vi "playback.vi"() -> ()   [LabVIEW 2012]
doc: "This VI will initialize the FPGA VI and read a user-defined number of samples from a DMA FIFO. When the data acquisition is complete this VI will read status information from the FPGA VI.\n\nFollow these instructions to run the VI.\n\n1. Select your RIO device from the dropdown.\n2. Set the sample period, number of samples to acquire per channel, and DMA block read size. \n\nNote: the block read size should be set to balance load on the host processor and the update rate of the user interface. A small block read size will update the user interface more often but will result in a higher load on the host processor."
uses:
  <vilib>/Analysis/3filter.llb/Butterworth Filter (DBL).vi
  <vilib>/Analysis/NI_AALBase.lvlib
  <vilib>/Analysis/NI_AALPro.lvlib
panel:
  in  "Filename":path=path "tdms"
  in  "Next Signal":bool
  in  "threshold ratio":dbl=3.0
  out "Sidemove":dbl
  out "Forward":dbl
  out "Threshold 3":dbl
  out "Threshold 2":dbl
  out "Threshold 1":dbl
  out "noise index":dbl[](array[numeric])
  out "Threshold 0":dbl
  out "Amplitude Spectrum":waveform(dbl)(graph)
  out "bad signal?":bool
  in  "Min Starting Index":i32=7000
  in  "Portion Duration":i32=1000
  out "amplitude 3":dbl
  out "amplitude 2":dbl
  out "amplitude 1":dbl
  out "amplitude 0":dbl
  in  "noise min":dbl=0.001
  out "Index 3":dbl
  out "Index 2":dbl
  out "Index 1":dbl
  out "Index 0":dbl
  in  "Send to ROS":bool
  out "ROS  Error":bool
  out "dt1":dbl
  out "dt2":dbl
  out "dt3":dbl
  out "pitch":dbl
  out "yaw":dbl
  out "z":dbl
  out "y":dbl
  out "x":dbl
  in  "Mode":T1(ring)=enum."Use Far Field"
  in  "Altitude":dbl=2.0
  in  "Display Filtered Signal":bool=TRUE
  out "Ratio at Index (%)":dbl
  out "Selected Index":i32
  in  "Threshold":dbl=0.1
  in  "low cutoff freq: fl":dbl=20000.0
  in  "high cutoff freq: fh":dbl=30000.0
  out "Yaw Chart":dbl(graph)
  out "Ch0 Signal":dbl[](graph)
  out "Extracted signal":dbl[][](graph)
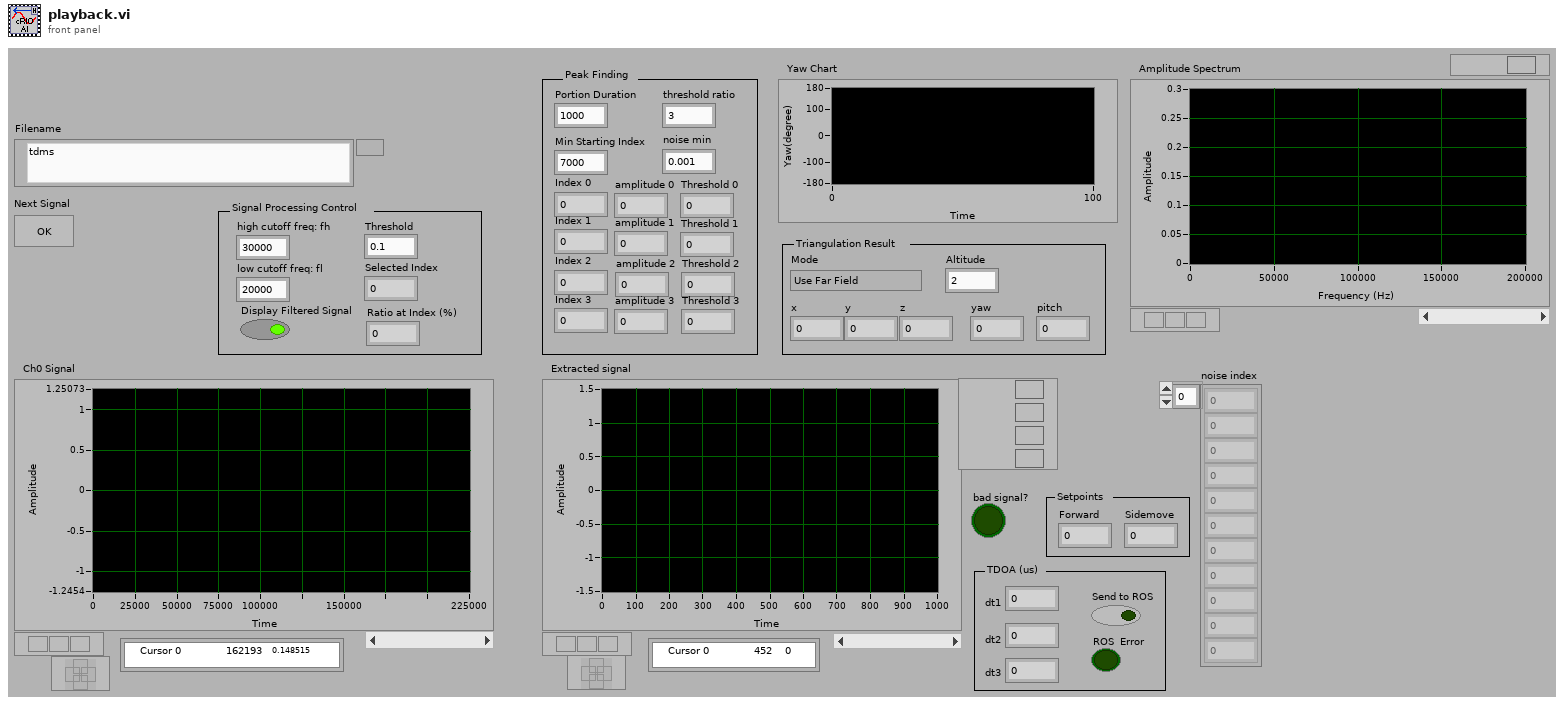
[diagram p1: front panel]
types:
  T1 = enum16{"Use Near Field", "Use Far Field", "Far Field with 3 hydrophones"}
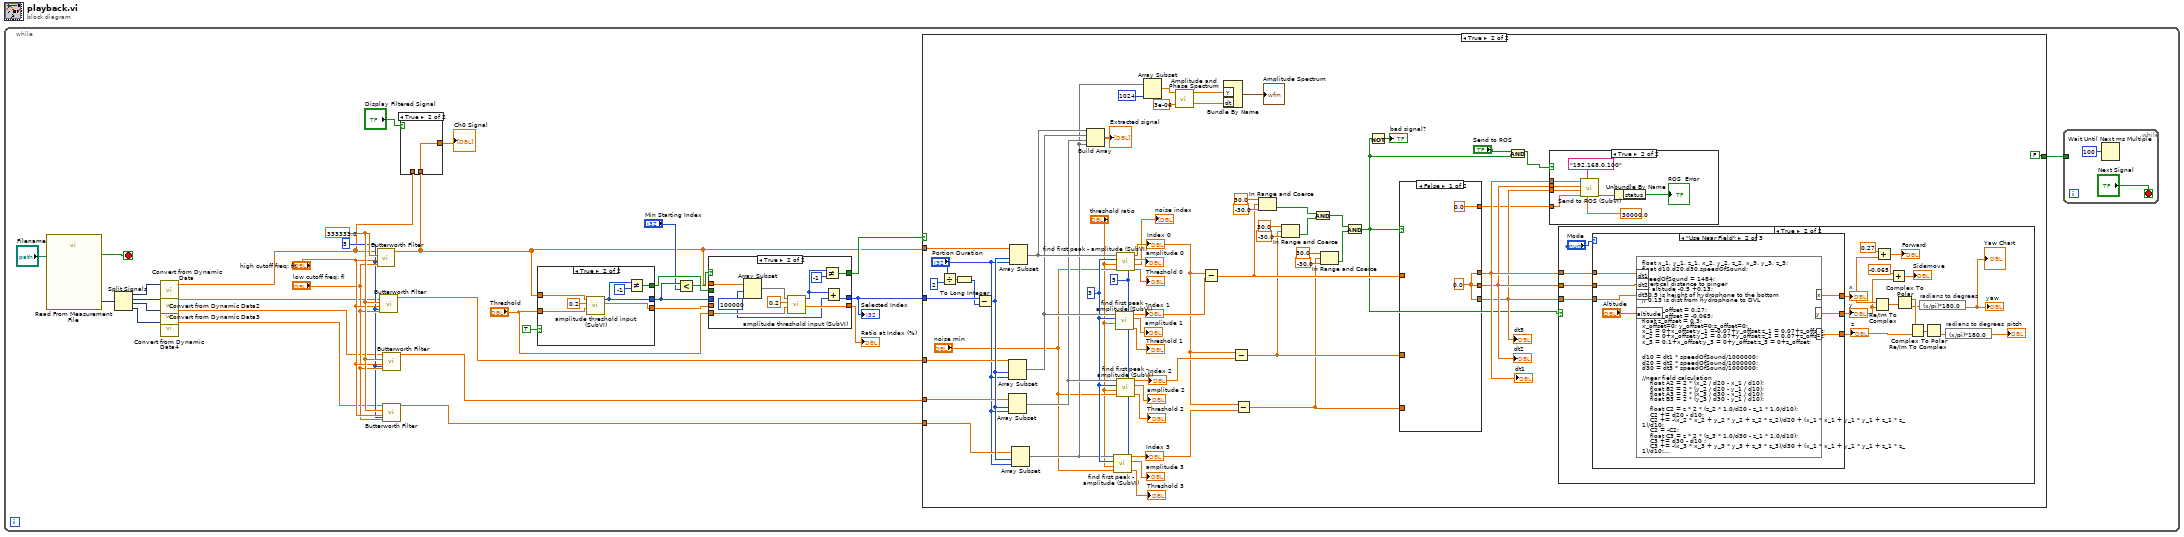
[diagram p0: block diagram]
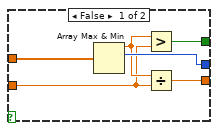
[diagram p4: hidden frame]
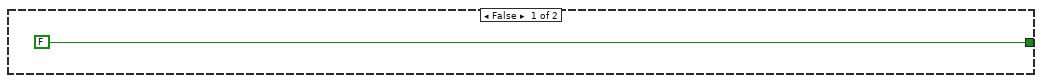
[diagram p5: hidden frame]
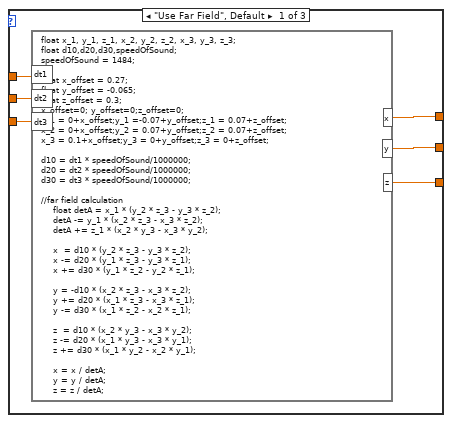
[diagram p7: hidden frame]
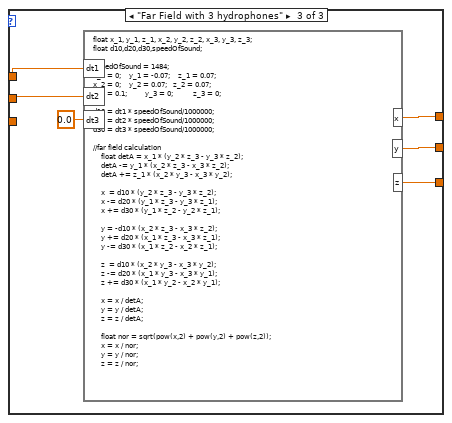
[diagram p8: hidden frame]
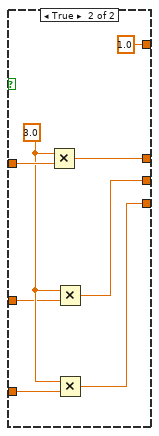
[diagram p10: hidden frame]
diagram:
  n1 = while {
    stop <- w5 stop-if-true
    w17 = 5
    w23 = 333333.0
    n2 = call "Read From Measurement File"("Filename"="Filename") -> ("Signals"=w10:dynamicdata, "EOF?"=w5:bool)  [unwired: 5 in, 4 out]
    n3 = Split Signals(w10) -> (w14:dynamicdata, w13:dynamicdata, w12:dynamicdata, w11:dynamicdata)  [unwired: 4 in]
    n4 = call "Convert from Dynamic Data"("Dynamic Data Type"=w14) -> ("Array"=w9:dbl[])  [unwired: 3 in]
    n5 = call "Convert from Dynamic Data2"("Dynamic Data Type"=w13) -> ("Array"=w8:dbl[])  [unwired: 3 in]
    n6 = call "Convert from Dynamic Data3"("Dynamic Data Type"=w12) -> ("Array"=w6:dbl[])  [unwired: 3 in]
    n7 = call "Convert from Dynamic Data4"("Dynamic Data Type"=w11) -> ("Array"=w7:dbl[])  [unwired: 3 in]
    n8 = call-poly <vilib>:"Butterworth Filter.vi"("order"=w17, "low cutoff freq: fl"="low cutoff freq: fl", "high cutoff freq: fh"="high cutoff freq: fh", "sampling freq: fs"=w23, "X"=w9) -> ("Filtered X"=w15:dbl[])  [unwired: 3 in, 1 out]
    n9 = call-poly <vilib>:"Butterworth Filter.vi"("order"=w17, "low cutoff freq: fl"="low cutoff freq: fl", "high cutoff freq: fh"="high cutoff freq: fh", "sampling freq: fs"=w23, "X"=w8) -> ("Filtered X"=w20:dbl[])  [unwired: 3 in, 1 out]
    n10 = call-poly <vilib>:"Butterworth Filter.vi"("order"=w17, "low cutoff freq: fl"="low cutoff freq: fl", "high cutoff freq: fh"="high cutoff freq: fh", "sampling freq: fs"=w23, "X"=w7) -> ("Filtered X"=w18:dbl[])  [unwired: 3 in, 1 out]
    n11 = call-poly <vilib>:"Butterworth Filter.vi"("order"=w17, "low cutoff freq: fl"="low cutoff freq: fl", "high cutoff freq: fh"="high cutoff freq: fh", "sampling freq: fs"=w23, "X"=w6) -> ("Filtered X"=w19:dbl[])  [unwired: 3 in, 1 out]
    n12 = case shown="True" "Display Filtered Signal" {
      tunnel: w9 -> [w35 _]
      tunnel: [w35 w36] -> w3
      tunnel: w15 -> [_ w36]
      frame False {
      }
      frame True {
      }
    }
    "Ch0 Signal" <- w3
    n13 = case shown="True" TRUE {
      tunnel: w15 -> [w55 w62]
      tunnel: [w52 w59] -> w29
      tunnel: [w53 w58] -> w26
      tunnel: [w54 w57] -> w31
      tunnel: "Threshold" -> [w50 w56]
      frame False {
        n14 = Array Max & Min(array=w55) -> (max value=w51:dbl, max index (indices)=w53:i32)  [unwired: 2 out]
        n15 = Greater?(x=w51, y=w50) -> (0:w54:bool)
        n16 = Divide(x=w51, y=w50) -> (x/y=w52:dbl)
      }
      frame True {
        n17 = call "amplitude threshold input (SubVI).vi"("threshold"=w56, "%max amplitude"=0.2, "Array"=w62) -> ("actual ratio (%)"=w59:dbl, "Index"=w58:i32)  [unwired: 7 in]
        n18 = Not Equal?(x=w58, y=-1) -> (x != y?=w57:bool)
      }
    }
    n19 = Less?(x=w26, y="Min Starting Index") -> (x < y?=w30:bool)
    n20 = case shown="True" w30 {
      tunnel: w31 -> [w39 _]
      tunnel: w29 -> [w37 _]
      tunnel: w15 -> [_ w49]
      tunnel: "Threshold" -> [_ w45]
      tunnel: [w39 w44] -> w24
      tunnel: [w38 w42] -> w25
      tunnel: [w37 w43] -> w27
      tunnel: w26 -> [w38 _]
      frame False {
      }
      frame True {
        w40 = 100000
        n21 = Array Subset(array=w49, index=w40) -> (w46:dbl[])  [unwired: 1 in]
        n22 = call "amplitude threshold input (SubVI).vi"("threshold"=w45, "%max amplitude"=0.2, "Array"=w46) -> ("actual ratio (%)"=w43:dbl, "Index"=w41:i32)  [unwired: 7 in]
        n23 = Not Equal?(x=w41, y=-1) -> (x != y?=w44:bool)
        n24 = Add(x=w41, y=w40) -> (x+y=w42:i32)
      }
    }
    "Ratio at Index (%)" <- w27
    "Selected Index" <- w25
    n25 = case shown="True" w24 {
      tunnel: w20 -> [_ w122]
      tunnel: w19 -> [_ w121]
      tunnel: w18 -> [_ w120]
      tunnel: w15 -> [_ w119]
      tunnel: w25 -> [_ w118]
      tunnel: [FALSE FALSE] -> w2
      frame False {
      }
      frame True {
        w71 = 5
        w84 = 3
        n26 = Divide(x="Portion Duration", y=2) -> (x/y=w115:dbl)
        n27 = To Long Integer(number=w115) -> (32bit integer=w114:i32)
        n28 = Subtract(x=w118, y=w114) -> (x-y=w123:i32)
        n29 = Array Subset(array=w121, index=w123, length="Portion Duration") -> (w85:dbl[])
        n30 = Array Subset(array=w122, index=w123, length="Portion Duration") -> (w89:dbl[])
        n31 = Array Subset(array=w119, index=w123, length="Portion Duration") -> (w91:dbl[])
        n32 = Array Subset(array=w120, index=w123, length="Portion Duration") -> (w83:dbl[])
        n33 = Build Array(w91, w89, w85, w83) -> (→"Extracted signal":dbl[][])
        n34 = call "find first peak - amplitude (SubVI).vi"("Noise length"=w71, "Noise min"="noise min", "threshold ratio"="threshold ratio", "width"=w84, "Array"=w83) -> ("Peak threshold"=→"Threshold 3":dbl, "peak amplitude"=→"amplitude 3":dbl, "Index"=w82:dbl)  [unwired: 2 in, 2 out]
        "Index 3" <- w82
        n35 = call "find first peak - amplitude (SubVI).vi"("Noise length"=w71, "threshold ratio"="threshold ratio", "width"=w84, "Array"=w89) -> ("Peak threshold"=→"Threshold 1":dbl, "peak amplitude"=→"amplitude 1":dbl, "Index"=w88:dbl)  [unwired: 3 in, 2 out]
        "Index 1" <- w88
        n36 = call "find first peak - amplitude (SubVI).vi"("Noise length"=w71, "Noise min"="noise min", "threshold ratio"="threshold ratio", "width"=w84, "Array"=w91) -> ("Peak threshold"=→"Threshold 0":dbl, "noise index"=→"noise index":dbl[], "peak amplitude"=→"amplitude 0":dbl, "Index"=w78:dbl)  [unwired: 2 in, 1 out]
        "Index 0" <- w78
        n37 = call "find first peak - amplitude (SubVI).vi"("Noise length"=w71, "Noise min"="noise min", "threshold ratio"="threshold ratio", "width"=w84, "Array"=w85) -> ("Peak threshold"=→"Threshold 2":dbl, "peak amplitude"=→"amplitude 2":dbl, "Index"=w86:dbl)  [unwired: 2 in, 2 out]
        "Index 2" <- w86
        n38 = Array Subset(array=w83, length=1024) -> (w67:dbl[])  [unwired: 1 in]
        n39 = call <vilib>:"Amplitude and Phase Spectrum.vi"("dt"=3e-06, "Signal (V)"=w67) -> ("df"=w64:dbl, "Amp Spectrum Mag (Vrms)"=w65:dbl[])  [unwired: 1 in, 1 out]
        n40 = Subtract(x=w78, y=w88) -> (x-y=w110:dbl)
        n41 = Bundle By Name("Y"=w65, "dt"=w64) -> (→"Amplitude Spectrum":waveform(dbl))  [unwired: 1 in]
        n42 = Subtract(x=w78, y=w86) -> (x-y=w107:dbl)
        n43 = Subtract(x=w78, y=w82) -> (x-y=w104:dbl)
        n44 = In Range and Coerce(upper limit=30.0, x=w110, lower limit=-30.0) -> (In Range?=w103:bool)  [unwired: 1 out]
        n45 = In Range and Coerce(upper limit=30.0, x=w107, lower limit=-30.0) -> (In Range?=w102:bool)  [unwired: 1 out]
        n46 = And(x=w103, y=w102) -> (x .and. y?=w101:bool)
        n47 = In Range and Coerce(upper limit=30.0, x=w104, lower limit=-30.0) -> (In Range?=w100:bool)  [unwired: 1 out]
        n48 = And(x=w101, y=w100) -> (x .and. y?=w92:bool)
        n49 = Not(x=w92) -> (.not. x?=→"bad signal?":bool)
        n50 = case shown="False" w92 {
          tunnel: w110 -> [_ w178]
          tunnel: w107 -> [_ w176]
          tunnel: w104 -> [_ w175]
          tunnel: [w169 w174] -> w97
          tunnel: [w169 w173] -> w96
          tunnel: [w169 w172] -> w95
          tunnel: [0.0 1.0] -> w94
          frame False {
            w169 = 0.0
          }
          frame True {
            w177 = 3.0
            n51 = Multiply(x=w177, y=w178) -> (x*y=w174:dbl)
            n52 = Multiply(x=w177, y=w176) -> (x*y=w173:dbl)
            n53 = Multiply(x=w177, y=w175) -> (x*y=w172:dbl)
          }
        }
        "dt1" <- w97
        "dt2" <- w96
        "dt3" <- w95
        n54 = And(x="Send to ROS", y=w92) -> (x .and. y?=w93:bool)
        n55 = case shown="True" w93 {
          tunnel: w97 -> [_ w164]
          tunnel: w96 -> [_ w163]
          tunnel: w95 -> [_ w162]
          tunnel: w94 -> [_ w161]
          frame False {
          }
          frame True {
            n56 = call "Send to ROS (SubVI).vi"("frequency"=30000.0, "ROS IP"="192.168.0.100", "Good signal?"=w161, "dt 3"=w162, "dt2"=w163, "dt 1"=w164) -> ("error out"=w167:errorcluster)  [unwired: 5 in]
            n57 = Unbundle By Name(w167) -> ("status"=→"ROS  Error":bool)
          }
        }
        n58 = case shown="True" w92 {
          tunnel: w97 -> [_ w132]
          tunnel: w96 -> [_ w131]
          tunnel: w95 -> [_ w130]
          frame False {
          }
          frame True {
            n59 = case shown="\"Use Near Field\"" "Mode" {
              tunnel: [w147 w154 w159] -> w129
              tunnel: [w146 w153 w158] -> w126
              tunnel: [w145 w152 w157] -> w136
              tunnel: w132 -> [w144 w150 w156]
              tunnel: w131 -> [w143 w149 w155]
              tunnel: w130 -> [w142 w148 _]
              frame "Use Far Field", Default {
                n60 = formula code="float x_1, y_1, z_1, x_2, y_2, z_2, x_3, y_3, z_3;\nfloat d10,d20,d30,speedOfSound;\nspeedOfSound = 1484;\n\nfloat x_offset = 0.27;\nfloat y_offset = -0.065;\nfloat z_offset = 0.3;\nx_offset=0; y_offset=0;z_offset=0;\nx_1 = 0+x_offset;y_1 =-0.07+y_offset;z_1 = 0.07+z_offset;\nx_2 = 0+x_offset;y_2 = 0.07+y_offset;z_2 = 0.07+z_offset;\nx_3 = 0.1+x_offset;y_3 = 0+y_offset;z_3 = 0+z_offset;\n\nd10 = dt1 * speedOfSound/1000000;\nd20 = dt2 * speedOfSound/1000000;\nd30 = dt3 * speedOfSound/1000000;\n\n//far field calculation\n    float detA = x_1 * (y_2 * z_3 - y_3 * z_2);\n    detA -= y_1 * (x_2 * z_3 - x_3 * z_2);\n    detA += z_1 * (x_2 * y_3 - x_3 * y_2);\n\n    x  = d10 * (y_2 * z_3 - y_3 * z_2);\n    x -= d20 * (y_1 * z_3 - y_3 * z_1);\n    x += d30 * (y_1 * z_2 - y_2 * z_1);\n\n    y = -d10 * (x_2 * z_3 - x_3 * z_2);\n    y += d20 * (x_1 * z_3 - x_3 * z_1);\n    y -= d30 * (x_1 * z_2 - x_2 * z_1);\n\n    z  = d10 * (x_2 * y_3 - x_3 * y_2);\n    z -= d20 * (x_1 * y_3 - x_3 * y_1);\n    z += d30 * (x_1 * y_2 - x_2 * y_1);\n\n    x = x / detA;\n    y = y / detA;\n    z = z / detA;\n\n    float nor = sqrt(pow(x,2) + pow(y,2) + pow(z,2));\n    x = x / nor;\n    y = y / nor;\n    z = z / nor;"("dt1"=w144, "dt2"=w143, "dt3"=w142) -> ("x"=w147:dbl, "y"=w146:dbl, "z"=w145:dbl)
              }
              frame "Use Near Field" {
                n61 = formula code="float x_1, y_1, z_1, x_2, y_2, z_2, x_3, y_3, z_3;\nfloat d10,d20,d30,speedOfSound;\n\nspeedOfSound = 1484;\n//vertical distance to pinger\nz= altitude -0.5 +0.13;\n// 0.5 is height of hydrophone to the bottom\n// 0.13 is dist from hydrophone to DVL\n\nfloat x_offset = 0.27;\nfloat y_offset = -0.065;\nfloat z_offset = 0.3;\nx_offset=0; y_offset=0;z_offset=0;\nx_1 = 0+x_offset;y_1 =-0.07+y_offset;z_1 = 0.07+z_offset;\nx_2 = 0+x_offset;y_2 = 0.07+y_offset;z_2 = 0.07+z_offset;\nx_3 = 0.1+x_offset;y_3 = 0+y_offset;z_3 = 0+z_offset;\n\n\nd10 = dt1 * speedOfSound/1000000;\nd20 = dt2 * speedOfSound/1000000;\nd30 = dt3 * speedOfSound/1000000;\n\n//near field calculation\n    float A2 = 2 * (x_2 / d20 - x_1 / d10);\n    float B2 = 2 * (y_2 / d20 - y_1 / d10);\n    float A3 = 2 * (x_3 / d30 - x_1 / d10);\n    float B3 = 2 * (y_3 / d30 - y_1 / d10);\n    \n    float C2 = z * 2 * (z_2 * 1.0/d20 - z_1 * 1.0/d10);\n    C2 += d20 - d10;\n    C2 += -(x_2 * x_2 + y_2 * y_2 + z_2 * z_2)/d20 + (x_1 * x_1 + y_1 * y_1 + z_1 * z_1)/d10;\n    C2 = -C2;\n    float C3 = z * 2 * (z_3 * 1.0/d30 - z_1 * 1.0/d10);\n    C3 += d30 - d10 ;\n    C3 += -(x_3 * x_3 + y_3 * y_3 + z_3 * z_3)/d30 + (x_1 * x_1 + y_1 * y_1 + z_1 * z_1)/d10;\n    C3 = -C3;\n\n    if (A2*B3 == A3*B2) {\n        x = 0;\n        y = 0;\n    }\n    else {\n        x = (C2 * B3 - C3 * B2) / (A2 * B3 - A3 * B2);\n        y = (C3 * A2 - C2 * A3) / (B3 * A2 - B2 * A3);\n    }"("dt1"=w150, "dt2"=w149, "dt3"=w148, "altitude"="Altitude") -> ("x"=w154:dbl, "y"=w153:dbl, "z"=w152:dbl)
              }
              frame "Far Field with 3 hydrophones" {
                n62 = formula code="float x_1, y_1, z_1, x_2, y_2, z_2, x_3, y_3, z_3;\nfloat d10,d20,d30,speedOfSound;\n\nspeedOfSound = 1484;\nx_1 = 0;    y_1 = -0.07;    z_1 = 0.07;\nx_2 = 0;    y_2 = 0.07;   z_2 = 0.07;\nx_3 = 0.1;         y_3 = 0;          z_3 = 0;\n\nd10 = dt1 * speedOfSound/1000000;\nd20 = dt2 * speedOfSound/1000000;\nd30 = dt3 * speedOfSound/1000000;\n\n//far field calculation\n    float detA = x_1 * (y_2 * z_3 - y_3 * z_2);\n    detA -= y_1 * (x_2 * z_3 - x_3 * z_2);\n    detA += z_1 * (x_2 * y_3 - x_3 * y_2);\n\n    x  = d10 * (y_2 * z_3 - y_3 * z_2);\n    x -= d20 * (y_1 * z_3 - y_3 * z_1);\n    x += d30 * (y_1 * z_2 - y_2 * z_1);\n\n    y = -d10 * (x_2 * z_3 - x_3 * z_2);\n    y += d20 * (x_1 * z_3 - x_3 * z_1);\n    y -= d30 * (x_1 * z_2 - x_2 * z_1);\n\n    z  = d10 * (x_2 * y_3 - x_3 * y_2);\n    z -= d20 * (x_1 * y_3 - x_3 * y_1);\n    z += d30 * (x_1 * y_2 - x_2 * y_1);\n\n    x = x / detA;\n    y = y / detA;\n    z = z / detA;\n\n    float nor = sqrt(pow(x,2) + pow(y,2) + pow(z,2));\n    x = x / nor;\n    y = y / nor;\n    z = z / nor;"("dt1"=w156, "dt2"=w155, "dt3"=0.0) -> ("x"=w159:dbl, "y"=w158:dbl, "z"=w157:dbl)
              }
            }
            "x" <- w129
            "y" <- w126
            "z" <- w136
            n63 = Re/Im To Complex(1:w126, 2:w129) -> (0:w134:cdb)
            n64 = Add(x=0.27, y=w129) -> (x+y=→"Forward":dbl)
            n65 = Add(x=-0.065, y=w126) -> (x+y=→"Sidemove":dbl)
            n66 = Complex To Polar(r * e^(i*theta)=w134) -> (r=w137:dbl, theta=w135:dbl)
            n67 = Re/Im To Complex(1:w136, 2:w137) -> (0:w138:cdb)
            n68 = expression code="(x/pi)*180.0"(w135) -> (→"yaw" →"Yaw Chart":dbl)
            n69 = Complex To Polar(r * e^(i*theta)=w138) -> (theta=w140:dbl)  [unwired: 1 out]
            n70 = expression code="(x/pi)*180.0"(w140) -> (→"pitch":dbl)
          }
        }
      }
    }
    n71 = while {
      tunnel: w2 -> [_]
      stop <- "Next Signal" stop-if-true
      n72 = Wait Until Next ms Multiple(millisecond multiple=u32 100) -> ()  [unwired: 1 out]
    }
  }
